vi "Read_type.vi"(8 "error in (no error)":errorcluster, 11 "PrepLinePictureObjects in":refnum<class "PrepLineObject.lvclass">) -> (0 "error out":errorcluster, 2 "type":string, 3 "PrepLinePictureObjects out":refnum<class "PrepLineObject.lvclass">)   [LabVIEW 2017, in "PrepLineObject.lvclass"]
doc: "gets the type of the PrepLine Picture Object (switch, pressure, temp)"
uses:
  PrepLineObject.lvclass
  PrepLineObject.lvclass/PrepLineObject.ctl
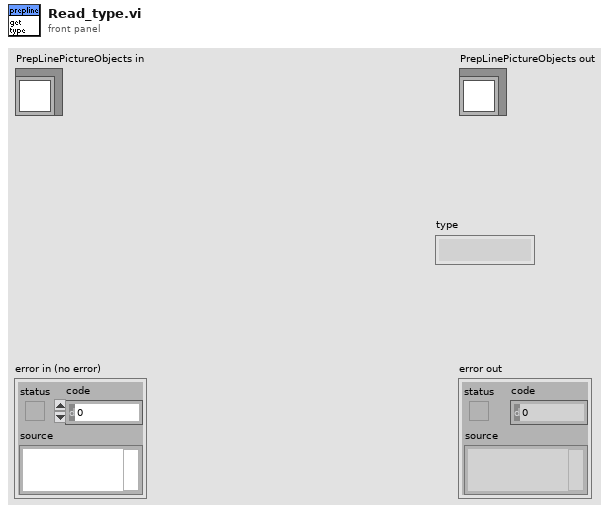
[diagram p1: front panel]
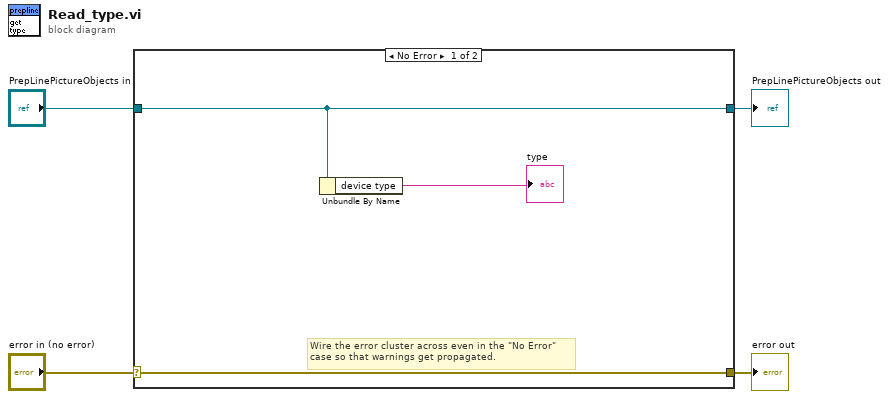
[diagram p0: block diagram]
diagram:
  n1 = case shown="No Error" "error in (no error)" {
    selector: "error in (no error)" -> [w7 w9]
    tunnel: [w7 w9] -> w3
    tunnel: [w6 w8] -> w1
    tunnel: "PrepLinePictureObjects in" -> [w6 w8]
    frame No Error {
      # "Wire the error cluster across even in the \"No Error\"\ncase so that warnings get propagated."
      n2 = Unbundle By Name(w6) -> ("device type"=→"type":string)
    }
    frame Error {
    }
  }
  "error out" <- w3
  "PrepLinePictureObjects out" <- w1
